vi "clear cancel dialog error.vi"(11 "error in":errorcluster caption="error in (no error)") -> (15 "error out":errorcluster)   [LabVIEW 2014]
doc: "This vi provides recovery from an error caused by cancelling the reload control parameters file dialog. The cancellation error is removed from the error bus so that the user can try the reload again. All other errors pass through unchanged.\n\nPaul K Dixon\nPhysics 350\nPaul K Dixon"
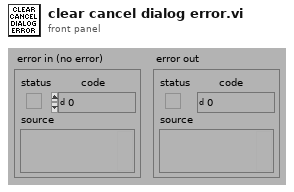
[diagram p1: front panel]
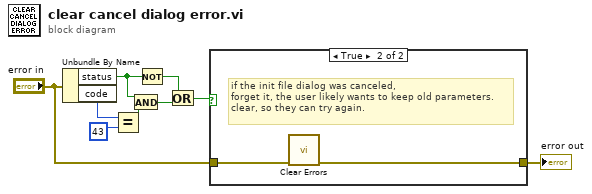
[diagram p0: block diagram]
diagram:
  n1 = Unbundle By Name("error in") -> ("status"=w5:bool, "code"=w7:i32)
  n2 = Equal?(x=w7, y=43) -> (x = y?=w6:bool)
  n3 = And(x=w5, y=w6) -> (x .and. y?=w9:bool)
  n4 = Not(x=w5) -> (.not. x?=w4:bool)
  n5 = Or(x=w4, y=w9) -> (x .or. y?=w3:bool)
  n6 = case shown="True" w3 {
    tunnel: [w10 w11] -> w1
    tunnel: "error in" -> [w10 w12]
    frame False {
      # "some other error, possibly from\nfile dialog. Bypass"
    }
    frame True {
      # "if the init file dialog was canceled,\nforget it, the user likely wants to keep old parameters.\nclear, so they can try again."
      n7 = call <vilib>:"Clear Errors.vi"("error in (no error)"=w12) -> ("error out"=w11:errorcluster)  [unwired: 1 in, 5 out]
    }
  }
  "error out" <- w1
